vi "MICS Impedance Measurement.vi"(7 "Test Current":enum16{"Low (200uA)", "High (500uA)"}(ring)=enum."High (500uA)", 8 "error in":errorcluster, 9 "Channel B":u8=2, 10 "Channel A":u8=1, 11 "VISA resource name in":refnum<visa-resource-name>) -> (0 "error out":errorcluster, 1 "Response Data":string, 2 "Text Out":string, 3 "Impedance (Ohms)":u16)   [LabVIEW 2020]
uses:
  Typedef Command List.ctl
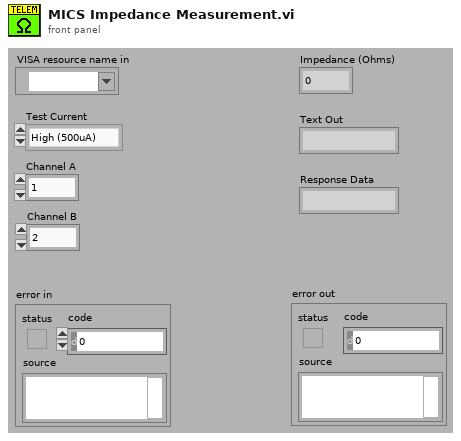
[diagram p1: front panel]
types:
  T1 = typedef "Typedef Command List.ctl" = enum16{"Get xPG Status", "xPG Stimulation", "Select Program", "Increment Program Amplitude", "Decrement Program Amplitude", "Get PoP Constants", "Get PPC Constants", "Get Program Names", "Set Pulse Amplitude", "Increment Pulse Amplitude", "Decrement Pulse Amplitude", "Get Pulse Widths", "Set Pulse Widths", "Increment Pulse Width", "Decrement Pulse Width", "Get Program Frequency", "Set Program Frequency", "Increment Program Frequency", "Decrement Program Frequency", "Inject Event", "Charging Control", "Get xPG Identity", "Set xPG Identity", "Restore Program Defaults", "Get Program Definition", "Set Program Definition", "Get Program Constants", "Set Program Constants", "Get Configurable Device Parameters", "Set Configurable Device Parameters", "Get Pulse Constants", "Set Pulse Constants", "Get Lead Limits", "Set Lead Limits", "Get Channel Calibrations", "Set Channel Calibrations", "<reserved 2>", "<reserved 3>", "<reserved 4>", "<reserved 5>", "<reserved 6>", "<reserved 7>", "Get Stim Asic HV Calibrations", "Set Stim Asic HV Calibrations", "<reserved 8>", "<reserved 9>", "Get CP Data", "Set CP Data", "Clear Log", "Read Log", "Append Log", "Get Patient Program Runtime", "Set Patient Program Runtime", "Impedance Measurement", "Enter Storage Mode", "Echo Short", "Echo Long", "Get General Calibration", "Set General Calibration", "Get Trim List", "Set Trim List", "Get Counter", "Set Counter", "Get Test Stimulation", "Set Test Stimulation", "Get Titration Stimulation", "Set Titration Stimulation", "Get Ramp Time", "Set Ramp Time", "Get VBAT", "Set Software Description Block", "Get Software Description Block", "Write Memory", "Read Memory", "Reset xPG", "Erase Flash Block", "Write Vectors", "Read Vectors", "Diagnostic Data", "Set Background Impedance", "Get Background Impedence ", "Set Test Waveform", "Calibrate Channel", "Get Log Range", "Reserved 0x55", "Reserved 0x56", "MICS Options", "Pair PPC", "Pair POP", "Stop Bootloader", "Tune MICS", "MICS Diagnostics", "Undefined"}
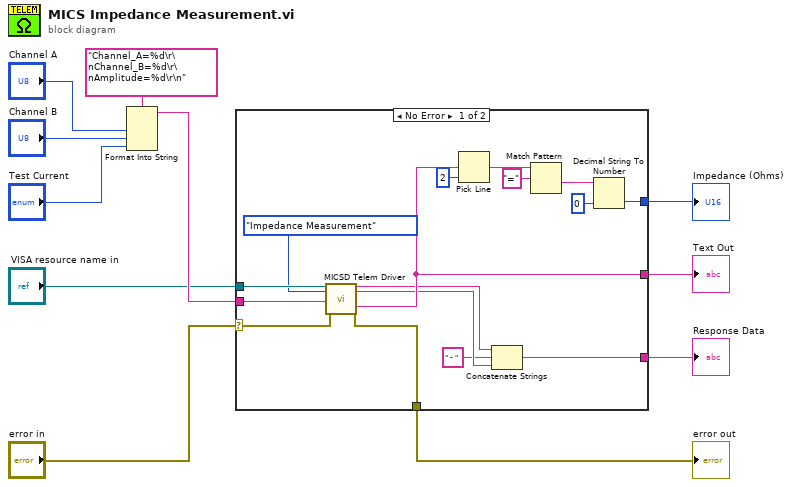
[diagram p0: block diagram]
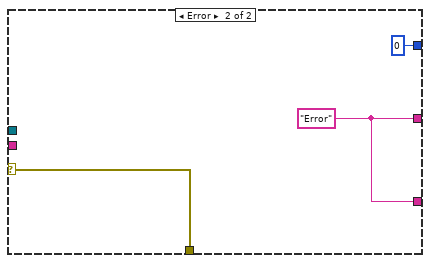
[diagram p2: hidden frame]
diagram:
  n1 = Format Into String(format string="Channel_A=%d\r\nChannel_B=%d\r\nAmplitude=%d\r\n", "Channel A", "Channel B", "Test Current") -> (resulting string=w9:string)  [unwired: 2 in, 1 out]
  n2 = case shown="No Error" "error in" {
    selector: "error in" -> [w12 w28]
    tunnel: [w27 w29] -> w11
    tunnel: w9 -> [w21 _]
    tunnel: "VISA resource name in" -> [w20 _]
    tunnel: [w19 w28] -> w4
    tunnel: [w16 w29] -> w3
    tunnel: [w13 u16 0] -> w2
    frame No Error {
      n3 = call "MICSD Telem Driver.vi"("VISA Resource Name"=w20, "Command"=Typedef_Command_List."Impedance Measurement", "Parameters"=w21, "error in (no error)"=w12) -> ("Response Token"=w17:string, "Response Code"=w18:string, "Data"=w27:string, "error out"=w19:errorcluster)  [unwired: 9 in, 3 out]
      n4 = Pick Line(multi-line string=w27, line index=2) -> (output string=w23:string)  [unwired: 1 in]
      n5 = Concatenate Strings(w17, " - ", w18) -> (w16:string)
      n6 = Match Pattern(string=w23, regular expression="=") -> (after substring=w25:string)  [unwired: 1 in, 3 out]
      n7 = Decimal String To Number(string=w25, default (0L)=u16 0 ("default (0 I32)")) -> (number=w13:u16)  [unwired: 1 in, 1 out]
    }
    frame Error {
      w29 = "Error" ("Data")
    }
  }
  "Text Out" <- w11
  "error out" <- w4
  "Response Data" <- w3
  "Impedance (Ohms)" <- w2
